vi "getElementFromVData.vi"(8 "error in (no error)":errorcluster, 9 "index Array 2":i32[](array[numeric]), 10 "Settings VData":variant[](array[variant]), 11 "Cluster in":variant) -> (0 "error out":errorcluster, 3 "element out":variant)   [LabVIEW 2011]
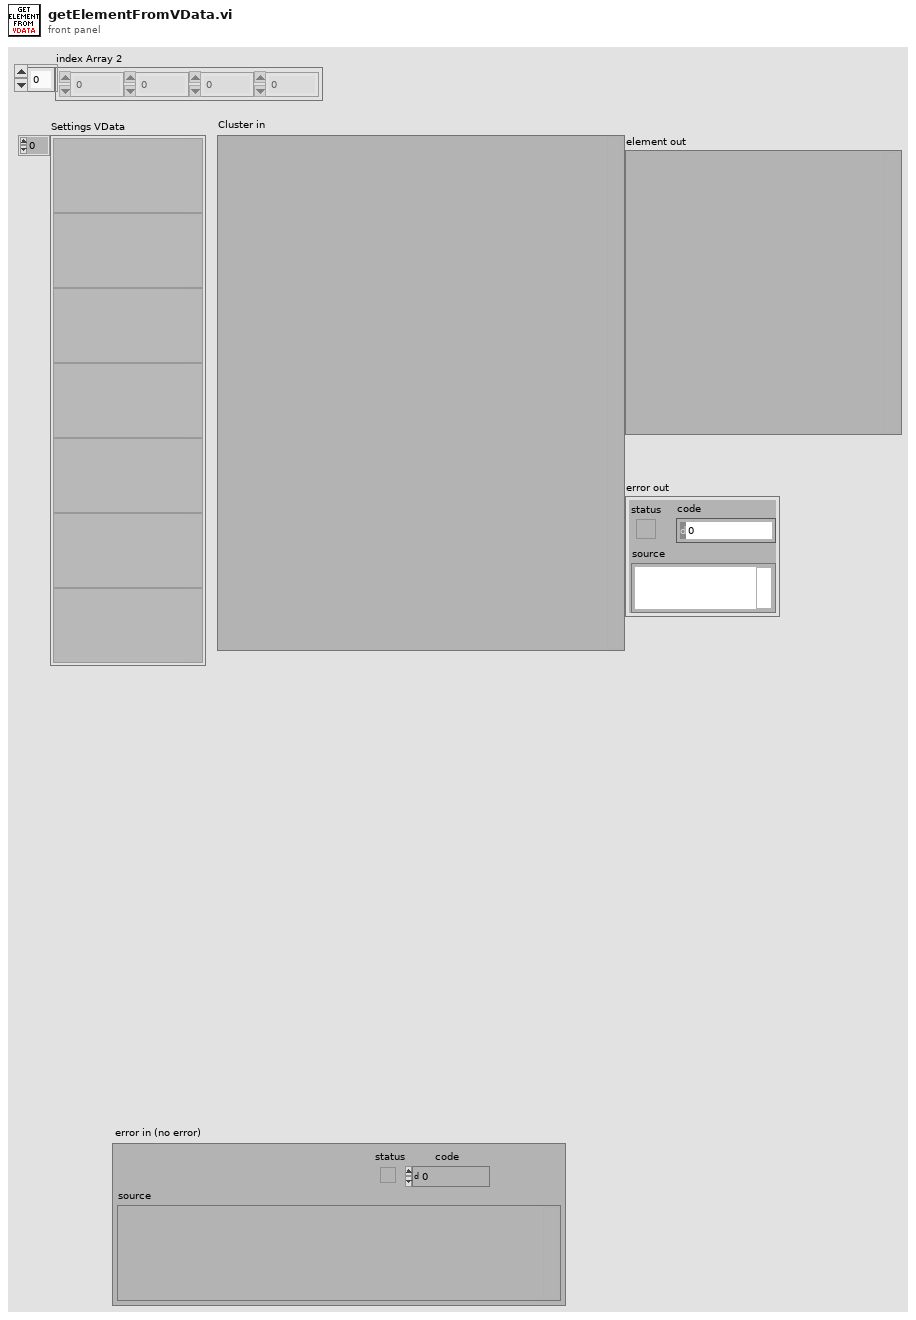
[diagram p1: front panel]
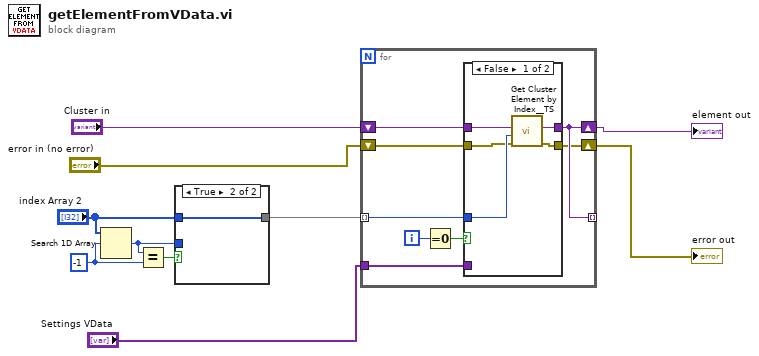
[diagram p0: block diagram]
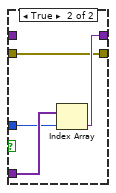
[diagram p2: hidden frame]
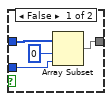
[diagram p3: hidden frame]
diagram:
  w8 = -1 ("element")
  n1 = Search 1D Array(1D array="index Array 2", element=w8) -> (index of element=w9:i32)  [unwired: 1 in]
  n2 = Equal?(x=w9, y=w8) -> (x = y?=w7:bool)
  n3 = case shown="True" w7 {
    tunnel: "index Array 2" -> [w14 w15]
    tunnel: w9 -> [w12 _]
    tunnel: [w11 w15] -> w3
    frame False {
      n4 = Array Subset(array=w14, index=0, length=w12) -> (w11:i32[])
    }
    frame True {
    }
  }
  n5 = for {
    tunnel: w3 -> [w22] mode=indexing
    shift-right: [w21] -> w1
    shift-left: "Cluster in" -> [w23]
    tunnel: [w21] -> _ mode=indexing
    shift-right: [w20] -> w2
    shift-left: "error in (no error)" -> [w19]
    tunnel: "Settings VData" -> [w17]
    i -> [w18]
    n6 = Equal To 0?(x=w18) -> (x = 0?=w16:bool)
    n7 = case shown="False" w16 {
      tunnel: w23 -> [w28 _]
      tunnel: w22 -> [w27 w31]
      tunnel: [w26 w30] -> w21
      tunnel: [w25 w29] -> w20
      tunnel: w19 -> [w24 w29]
      tunnel: w17 -> [_ w32]
      frame False {
        n8 = call "Get Cluster Element by Index__TS.vi"("error in (no error)"=w24, "index of element"=w27, "Cluster"=w28) -> ("error out"=w25:errorcluster, "VElement"=w26:variant)  [unwired: 6 in, 1 out]
      }
      frame True {
        n9 = Index Array(array=w32, index=w31) -> (element=w30:variant)
      }
    }
  }
  "element out" <- w1
  "error out" <- w2
